vi "ProdaNG.Configurator.Glb.Write.vi"(7 "DB":T1, 8 "error in (no error)":errorcluster) -> (0 "error out":errorcluster)   [LabVIEW 2016]
uses:
  ProdaNG.Configurator.DB.ctl
  Tools/Tma.lib/nlconfig.llb/fp2ini mode.ctl
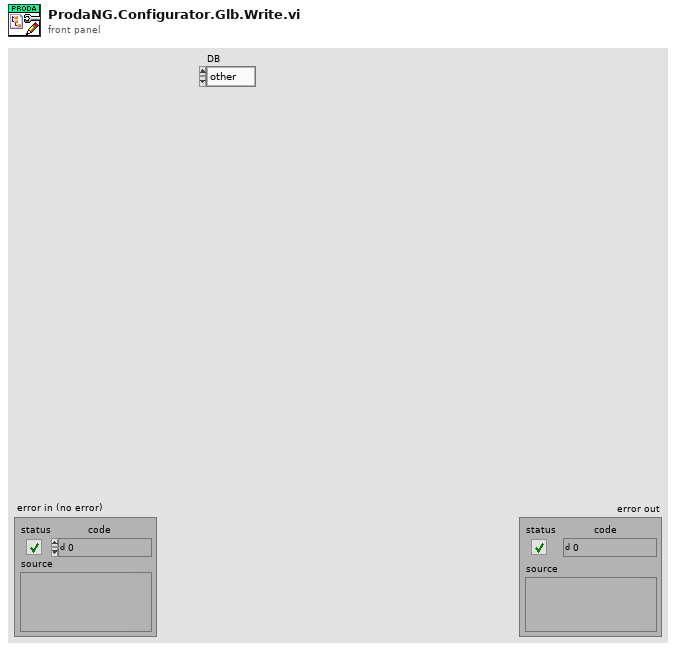
[diagram p1: front panel]
types:
  T1 = typedef "ProdaNG.Configurator.DB.ctl" = enum16{"other", "WPL", "WPK"}
  T2 = typedef "fp2ini mode.ctl" = enum16{"Read Controls", "Write Controls", "Write Indicators", "Read Indicators", "Write all", "Read all"}
  T3 = enum32{"invalid app kind", "Development System", "Run Time System", "Student Edition", "Embedded LabVIEW", "Evaluation", "Custom"}
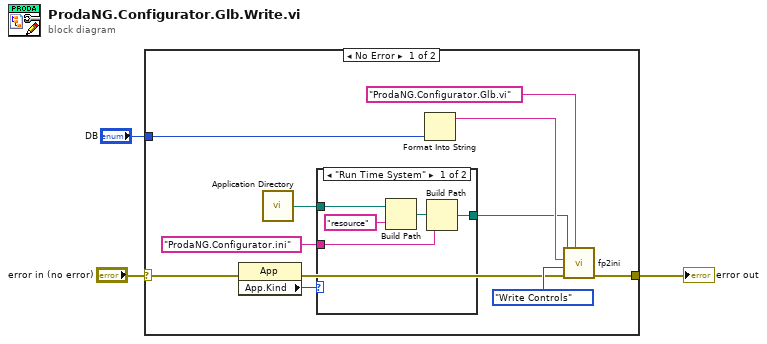
[diagram p0: block diagram]
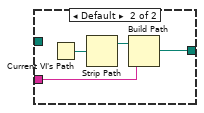
[diagram p2: hidden frame]
diagram:
  n1 = case shown="No Error" "error in (no error)" {
    selector: "error in (no error)" -> [w6 w24]
    tunnel: [w11 w24] -> w2
    tunnel: "DB" -> [w13 _]
    frame No Error {
      n2 = property class="App"(error in=w6) -> (error out=w5:errorcluster, "App.Kind"=w8:T3)  [unwired: 1 in, 1 out]
      n3 = call <vilib>:"Application Directory.vi"() -> ("Application Directory"=w7:path)
      n4 = case shown="\"Run Time System\"" w8 {
        tunnel: [w19 w21] -> w4
        tunnel: "ProdaNG.Configurator.ini" ("name or relative path") -> [w18 w20]
        tunnel: w7 -> [w16 _]
        frame "Run Time System" {
          n5 = Build Path(base path=w16, name or relative path="resource") -> (appended path=w15:path)
          n6 = Build Path(base path=w15, name or relative path=w18) -> (appended path=w19:path)
        }
        frame Default {
          n7 = Current VI's Path() -> (path=w23:path)
          n8 = Strip Path(path=w23) -> (stripped path=w22:path)  [unwired: 1 out]
          n9 = Build Path(base path=w22, name or relative path=w20) -> (appended path=w21:path)
        }
      }
      n10 = Format Into String(w13) -> (resulting string=w12:string)  [unwired: 3 in, 1 out]
      n11 = call "fp2ini.vi"("vi-name (caller if empty)"="ProdaNG.Configurator.Glb.vi" ("name or relative path"), "error in"=w5, "mode"=fp2ini_mode."Write Controls", "section"=w12, "ini-file path"=w4) -> ("error out"=w11:errorcluster)  [unwired: 6 in]
    }
    frame Error {
    }
  }
  "error out" <- w2
